vi "State Queue MERGE.vi"(8 "error in (no error)":errorcluster, 10 "State que 2 in":T1[](array[typedef]), 11 "State que 1 in":T1[](array[typedef])) -> (0 "error out":errorcluster, 3 "State que out":T1[](array[typedef]))   [LabVIEW 2009, in "State Machine Lib.lvlib"]
doc: "Merges Q1 and !2 and returns the concatinated queues"
uses:
  State Machine Lib.lvlib
  STATE cluster.ctl
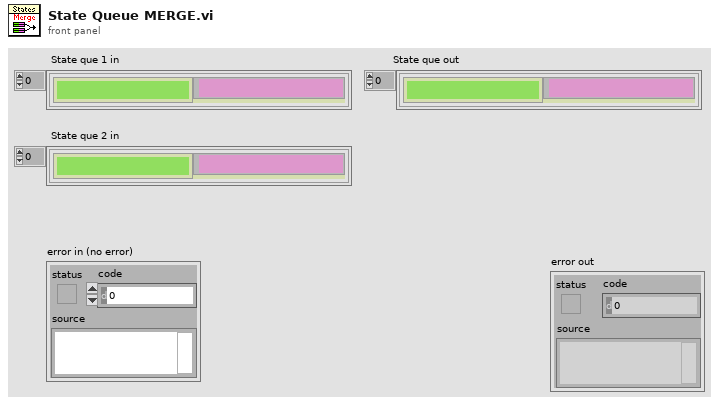
[diagram p1: front panel]
types:
  T1 = typedef "State Machine Lib.lvlib/STATE cluster.ctl" = cluster{"State":string, "Parameters":variant}
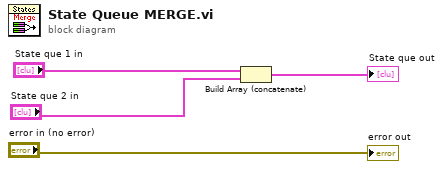
[diagram p0: block diagram]
diagram:
  n1 = Build Array (concatenate)("State que 1 in", "State que 2 in") -> (→"State que out":T1[])
  "error out" <- "error in (no error)"
